vi "05-Vending3_QSM.vi"() -> ()   [LabVIEW 2017]
uses:
  Support/03-Typedef.ctl
panel:
  in  "Change":bool
  in  "100 Yen":bool
  in  "Vend":bool
  in  "stop":bool
  out "Current Value":i32
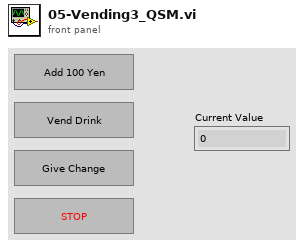
[diagram p1: front panel]
types:
  T1 = typedef "03-Typedef.ctl" = enum16{"Init", "Vend", "Change", "Add Money", "Idle", "Exit"}
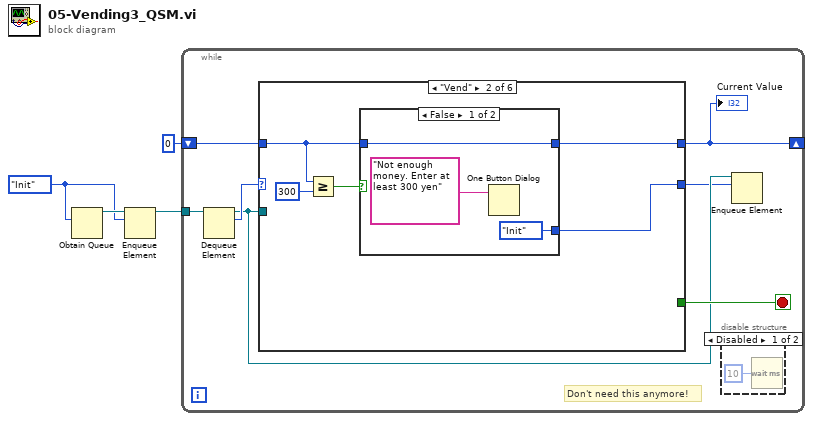
[diagram p0: block diagram]
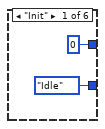
[diagram p3: hidden frame]
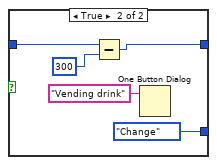
[diagram p4: hidden frame]
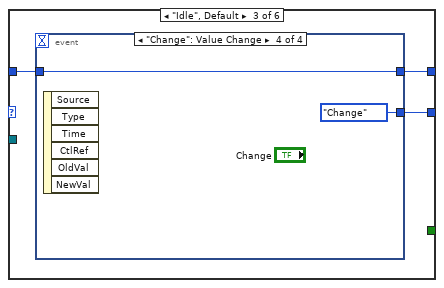
[diagram p5: hidden frame]
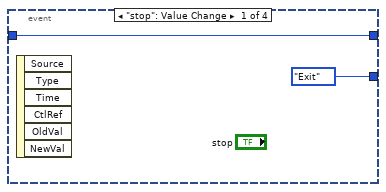
[diagram p6: hidden frame]
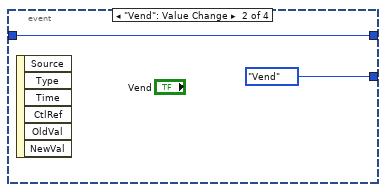
[diagram p7: hidden frame]
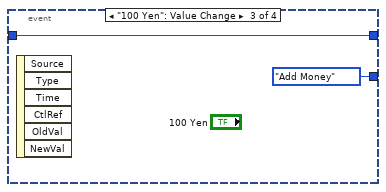
[diagram p8: hidden frame]
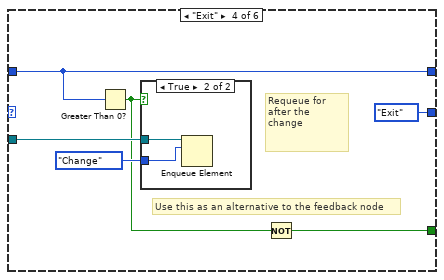
[diagram p9: hidden frame]
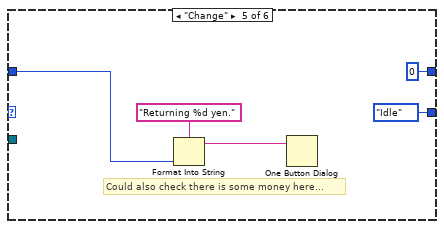
[diagram p11: hidden frame]
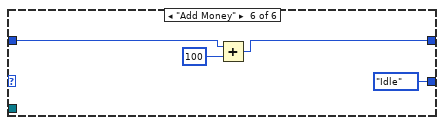
[diagram p12: hidden frame]
diagram:
  w2 = 03-Typedef."Init" ("Enum")
  n1 = Obtain Queue(element data type=w2) -> (queue out=w3:refnum<queue>)  [unwired: 4 in, 2 out]
  n2 = Enqueue Element(queue=w3, element=w2) -> (queue out=w1:refnum<queue>)  [unwired: 2 in, 2 out]
  n3 = while {
    shift-right: [w9] -> _
    shift-left: 0 -> [w10]
    tunnel: w1 -> [w8]
    stop <- w11 stop-if-true
    # "Don't need this anymore!"
    n4 = Dequeue Element(queue=w8) -> (queue out=w6:refnum<queue>, element=w7:T1)  [unwired: 2 in, 2 out]
    n5 = case shown="\"Vend\"" w7 {
      tunnel: [_ _ _ w39 _ _] -> w11
      tunnel: [03-Typedef."Idle" ("Enum") w15 w30 03-Typedef."Exit" ("Enum") 03-Typedef."Idle" ("Enum") 03-Typedef."Idle" ("Enum")] -> w5
      tunnel: w10 -> [_ w17 w29 w43 w48 w55]
      tunnel: [0 w16 w28 w43 0 w54] -> w9
      tunnel: w6 -> [_ _ _ w42 _ _]
      frame "Init" {
      }
      frame "Vend" {
        n6 = Greater Or Equal?(x=w17, y=300) -> (x >= y?=w18:bool)
        n7 = case shown="False" w18 {
          tunnel: w17 -> [w21 w26]
          tunnel: [w21 w24] -> w16
          tunnel: [03-Typedef."Init" ("Enum") 03-Typedef."Change" ("Enum")] -> w15
          frame False {
            n8 = One Button Dialog(message="Not enough money. Enter at least 300 yen") -> ()  [unwired: 1 in, 1 out]
          }
          frame True {
            n9 = Subtract(x=w26, y=300) -> (x-y=w24:i32)
            n10 = One Button Dialog(message="Vending drink") -> ()  [unwired: 1 in, 1 out]
          }
        }
      }
      frame "Idle", Default {
        n11 = event shown="[3] \"Change\": Value Change" {
          selector: _ -> [_ _ _ _]
          dyn-events: _ -> [_ _ _ _]
          timeout: _ -> [_ _ _ _]
          tunnel: [03-Typedef."Exit" ("t") 03-Typedef."Vend" ("Enum") 03-Typedef."Add Money" ("Enum") 03-Typedef."Change" ("Enum")] -> w30
          tunnel: w29 -> [w31 w33 w35 w38]
          tunnel: [w31 w33 w35 w38] -> w28
          event "stop": Value Change {
            n12 = event-data() -> ()  [unwired: 1 in, 6 out]
          }
          event "Vend": Value Change {
            n13 = event-data() -> ()  [unwired: 1 in, 6 out]
          }
          event "100 Yen": Value Change {
            n14 = event-data() -> ()  [unwired: 1 in, 6 out]
          }
          event "Change": Value Change {
            n15 = event-data() -> ()  [unwired: 1 in, 6 out]
          }
        }
      }
      frame "Exit" {
        # "Use this as an alternative to the feedback node"
        # "Requeue for after the change"
        n16 = Greater Than 0?(x=w43) -> (x > 0?=w40:bool)
        n17 = case shown="True" w40 {
          tunnel: w42 -> [_ w46]
          tunnel: 03-Typedef."Change" ("Enum") -> [_ w45]
          frame False {
          }
          frame True {
            n18 = Enqueue Element(queue=w46, element=w45) -> ()  [unwired: 2 in, 3 out]
          }
        }
        n19 = Not(x=w40) -> (.not. x?=w39:bool)
      }
      frame "Change" {
        # "Could also check there is some money here..."
        n20 = Format Into String(format string="Returning %d yen.", w48) -> (resulting string=w50:string)  [unwired: 2 in, 1 out]
        n21 = One Button Dialog(message=w50) -> ()  [unwired: 1 in, 1 out]
      }
      frame "Add Money" {
        n22 = Add(x=w55, y=100) -> (x+y=w54:i32)
      }
    }
    "Current Value" <- w9
    n23 = disable-structure shown="Disabled" {
      frame Disabled {
        n24 = Wait (ms)(milliseconds to wait=u32 10) -> ()  [unwired: 1 out]
      }
      frame Enabled {
      }
    }
    n25 = Enqueue Element(queue=w6, element=w5) -> ()  [unwired: 2 in, 3 out]
  }
